vi "Shoot.vi"   [LabVIEW 2017]
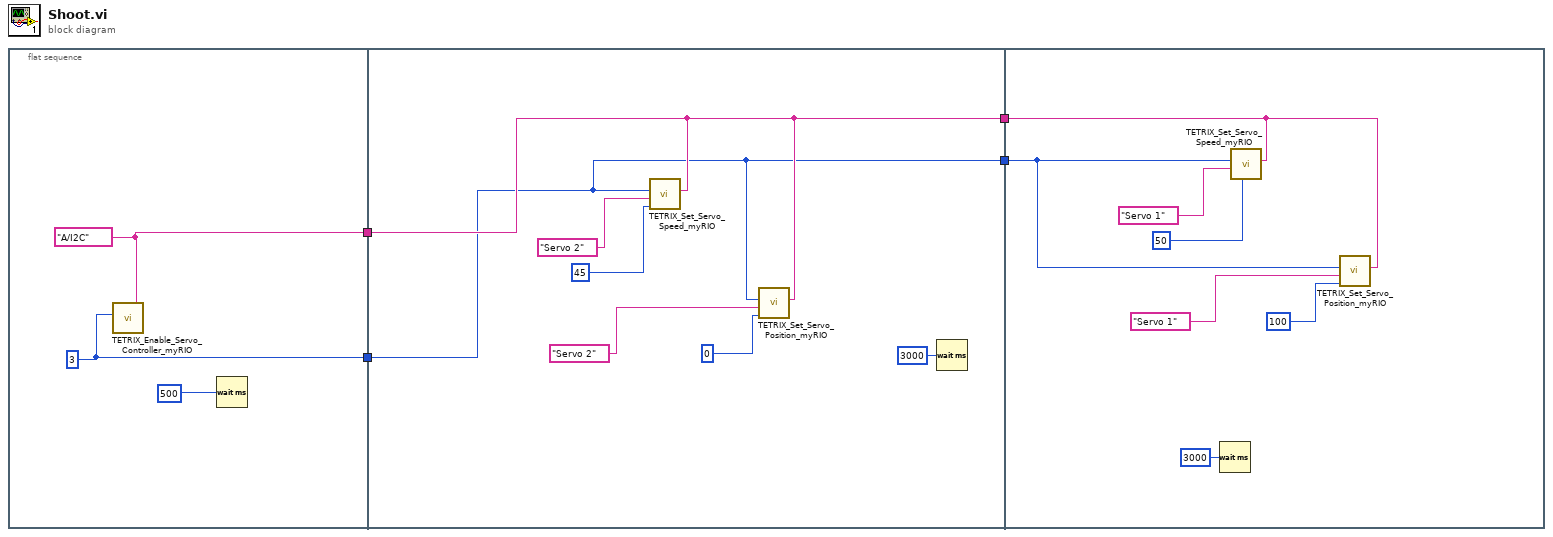
[diagram p0: block diagram]
diagram:
  n1 = flat-sequence {
    tunnel: [w6] -> w4
    tunnel: [w5] -> w3
    tunnel: w4 -> [w9]
    tunnel: w3 -> [w8]
    tunnel: [w9] -> w2
    tunnel: [w8] -> w1
    tunnel: w2 -> [w16]
    tunnel: w1 -> [w15]
    frame #0 {
      w5 = u8 3 ("Controller ID#  (I2C Address)")
      w6 = tag "A/I2C" ("myRIO MXP Port A/B")
      n2 = call <vilib>:"TETRIX_Enable_Servo_Controller_myRIO.vi"("myRIO MXP Port A/B"=w6, "Controller ID#  (I2C Address)"=w5) -> ()  [unwired: 5 in, 1 out]
      n3 = Wait (ms)(milliseconds to wait=u32 500 ("millisecond timer value")) -> ()  [unwired: 1 out]
    }
    frame #1 {
      n4 = call <vilib>:"TETRIX_Set_Servo_Speed_myRIO.vi"("myRIO MXP Port A/B"=w9, "Set Servo Speed (0 - 100 percent)"=u8 45, "Select Channel"="Servo 2", "Controller ID#  (I2C Address)"=w8) -> ()  [unwired: 3 in, 1 out]
      n5 = call <vilib>:"TETRIX_Set_Servo_Position_myRIO.vi"("myRIO MXP Port A/B"=w9, "Set Servo Position (0 - 180 degrees)"=u8 0, "Select Channel"="Servo 2", "Controller ID#  (I2C Address)"=w8) -> ()  [unwired: 3 in, 1 out]
      n6 = Wait (ms)(milliseconds to wait=u32 3000) -> ()  [unwired: 1 out]
    }
    frame #2 {
      n7 = Wait (ms)(milliseconds to wait=u32 3000) -> ()  [unwired: 1 out]
      n8 = call <vilib>:"TETRIX_Set_Servo_Speed_myRIO.vi"("myRIO MXP Port A/B"=w16, "Set Servo Speed (0 - 100 percent)"=u8 50, "Select Channel"="Servo 1", "Controller ID#  (I2C Address)"=w15) -> ()  [unwired: 3 in, 1 out]
      n9 = call <vilib>:"TETRIX_Set_Servo_Position_myRIO.vi"("myRIO MXP Port A/B"=w16, "Set Servo Position (0 - 180 degrees)"=u8 100, "Select Channel"="Servo 1", "Controller ID#  (I2C Address)"=w15) -> ()  [unwired: 3 in, 1 out]
    }
  }
